vi "DetectGreenPaper.vi"(8 "error in":errorcluster, 11 "Image In":T1) -> (0 "error out":errorcluster, 2 "Number of Matches (Color Location 1)":i32, 3 "Image Out":T1)   [LabVIEW 2013]
uses:
  <vilib>/vision/Image Controls.llb/IMAQ Image.ctl
  <vilib>/vision/NI_Vision_Development_Module.lvlib
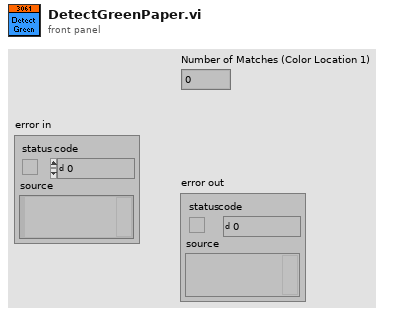
[diagram p1: front panel]
types:
  T1 = typedef "IMAQ Image.ctl" = refnum<image>
  T2 = typedef "Image Type" = u32
  T3 = cluster{"Global Rectangle":i32[], "Contours":cluster{"ID":enum32{"External", "Internal"}, "Type":u32, "Coordinates":i32[]}[]}
  T4 = cluster{"Position":cluster{"x":sgl, "y":sgl}, "Angle":sgl, "Scale":sgl, "Score":sgl, "Bounding Box":cluster{"x":sgl, "y":sgl}[]}[]
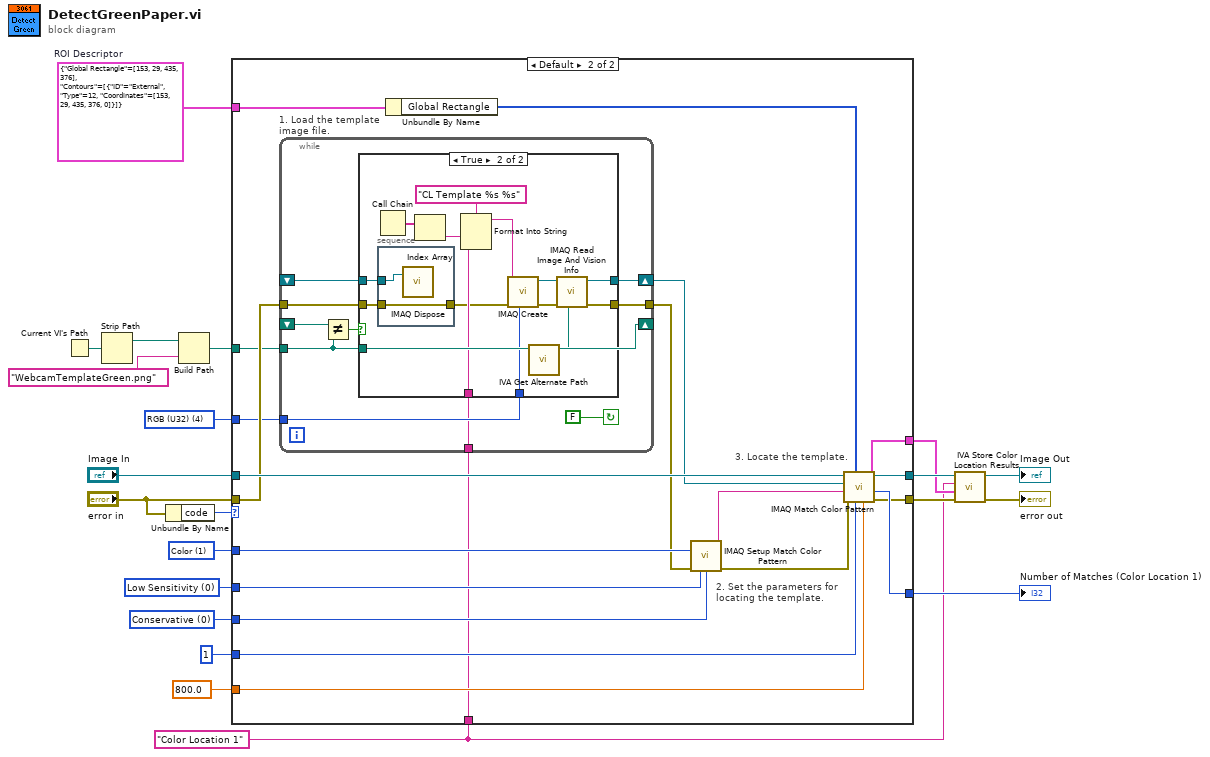
[diagram p0: block diagram]
diagram:
  w5 = "Color Location 1" ("Step Name")
  w14 = T2 4 items=["Grayscale (U8)", "Grayscale (I16)", "Grayscale (SGL)", "Complex (CSG)", "RGB (U32)", "HSL (U32)", "RGB (U64)"] ("Image Type")
  w15 = u32 0 items=["Conservative", "Balance", "Aggressive", "Very Aggressive"] ("Search Strategy")
  w16 = u32 0 items=["Low Sensitivity", "Medium Sensitivity", "High Sensitivity"] ("Color Sensitivity")
  w17 = u32 1 items=["Color and Shape", "Color", "Shape"] ("Match Feature Mode")
  w13 = T3 {"Global Rectangle"=[153, 29, 435, 376], "Contours"=[{"ID"=enum."External", "Type"=12, "Coordinates"=[153, 29, 435, 376, 0]}]}  # ROI Descriptor
  n1 = Current VI's Path() -> (path=w4:path)
  n2 = Strip Path(path=w4) -> (stripped path=w3:path)  [unwired: 1 out]
  n3 = Unbundle By Name("error in") -> ("code"=w11:i32)
  n4 = Build Path(base path=w3, name or relative path="WebcamTemplateGreen.png") -> (appended path=w1:path)
  n5 = case shown="Default" w11 {
    tunnel: sgl 800.0 ("Minimum Match Score") -> [_ w41]
    tunnel: 1 ("Number of Matches Requested") -> [_ w40]
    tunnel: [_ w39] -> w18
    tunnel: w17 -> [_ w38]
    tunnel: w16 -> [_ w37]
    tunnel: w15 -> [_ w36]
    tunnel: w1 -> [_ w28]
    tunnel: w14 -> [_ w27]
    tunnel: "error in" -> [_ w29]
    tunnel: w13 -> [_ w33]
    tunnel: [_ w31] -> w6
    tunnel: "Image In" -> [w22 w30]
    tunnel: [w22 w30] -> w7
    tunnel: [_ w24] -> w9
    tunnel: w5 -> [_ w23]
    frame -1074396199, -1074396198 {
      # "Discard Coordinate System Error"
    }
    frame Default {
      # "3. Locate the template."
      # "2. Set the parameters for\nlocating the template."
      n6 = while "1. Load the template image file." {
        shift-right: [w51] -> w26
        shift-left: _ -> [w50]
        tunnel: [w48] -> w25
        tunnel: w29 -> [w47]
        tunnel: w28 -> [w42]
        tunnel: w27 -> [w46]
        tunnel: w23 -> [w45]
        shift-right: [w42] -> _
        shift-left: _ -> [w44]
        stop <- FALSE continue-if-true
        n7 = Not Equal?(x=w44, y=w42) -> (x != y?=w43:bool)
        n8 = case shown="True" w43 {
          tunnel: [w53 w66] -> w51
          tunnel: w50 -> [w53 w58]
          tunnel: [w52 w63] -> w48
          tunnel: w47 -> [w52 w57]
          tunnel: w46 -> [_ w62]
          tunnel: w45 -> [_ w59]
          tunnel: w42 -> [_ w55]
          frame False {
          }
          frame True {
            n9 = Call Chain() -> (call chain=w61:string[])
            n10 = stacked-sequence {
              tunnel: w58 -> [w70]
              tunnel: w57 -> [w69]
              tunnel: [w69] -> w56
              frame #0 {
                n11 = call "IMAQ Dispose"("Image"=w70) -> ()  [unwired: 2 in, 4 out]
              }
            }
            n12 = Index Array(array=w61) -> (element=w60:string)  [unwired: 1 in]
            n13 = Format Into String(format string="CL Template %s %s" ("Image Name"), w60, w59) -> (resulting string=w68:string)  [unwired: 2 in, 1 out]
            n14 = call "IMAQ Create"("Image Name"=w68, "Image Type"=w62, "error in (no error)"=w56) -> ("New Image"=w65:T1, "error out"=w64:errorcluster)  [unwired: 1 in, 1 out]
            n15 = call <vilib>:"IVA Get Alternate Path.vi"("Path In"=w55) -> ("Path Out"=w54:path)  [unwired: 10 out]
            n16 = call "IMAQ Read Image And Vision Info"("File Path"=w54, "error in (no error)"=w64, "Image"=w65) -> ("error out"=w63:errorcluster, "Image Out"=w66:T1)  [unwired: 1 in, 6 out]
          }
        }
      }
      n17 = Unbundle By Name(w33) -> ("Global Rectangle"=w32:i32[])
      n18 = call "IMAQ Setup Match Color Pattern"("Match Feature Mode"=w38, "error in (no error)"=w25, "Color Sensitivity"=w37, "Search Strategy"=w36) -> ("Match Color Pattern Setup Data"=w35:string, "error out"=w34:errorcluster)  [unwired: 5 in, 5 out]
      n19 = call "IMAQ Match Color Pattern"("Minimum Match Score"=w41, "Number of Matches Requested"=w40, "Optional Rectangle"=w32, "error in (no error)"=w34, "Match Color Pattern Setup Data"=w35, "Template Image"=w26, "Image"=w30) -> ("error out"=w24:errorcluster, "Number of Matches"=w39:i32, "Matches"=w31:T4)  [unwired: 2 out]
    }
  }
  "Number of Matches (Color Location 1)" <- w18
  n20 = call <vilib>:"IVA Store Color Location Results.vi"("error in (no error)"=w9, "Matches"=w6, "Step Name"=w5, "Image in"=w7) -> ("error out"=→"error out":errorcluster, "Image dup"=→"Image Out":T1)  [unwired: 6 out]
